vi "Read Output.vi"(0 "VISA resource name":refnum<visa-resource-name>, 7 "Reading Source (T:Voltage)":bool=TRUE, 11 "error in (no error)":errorcluster) -> (4 "VISA resource name out":refnum<visa-resource-name>, 8 "Display Reading":dbl format="%^.4e", 15 "error out":errorcluster)   [LabVIEW 2020, in "Stanford Research PS300 Series.lvlib"]
doc: "This VI reads and displays the current value that is being outputted by the instrument."
uses:
  Stanford Research PS300 Series.lvlib
panel:
  # "Voltage \nCurrent"
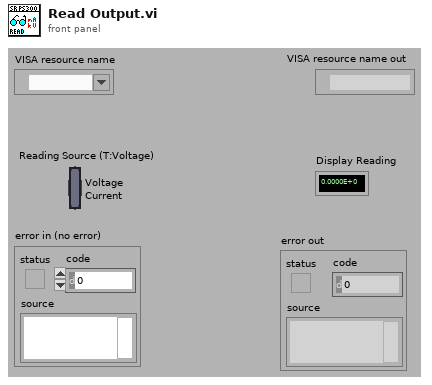
[diagram p1: front panel]
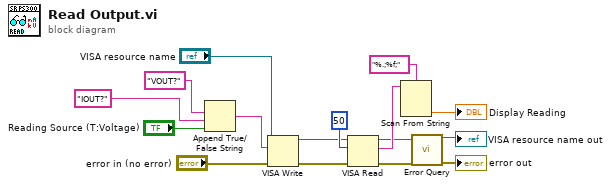
[diagram p0: block diagram]
diagram:
  n1 = Append True/False String(1:"Reading Source (T:Voltage)", 2:"IOUT?" ("false string"), 3:"VOUT?" ("true string")) -> (0:w10:string)  [unwired: 1 in]
  n2 = VISA Write(VISA resource name="VISA resource name", write buffer=w10, error in (no error)="error in (no error)") -> (VISA resource name out=w8:refnum<visa-resource-name>, error out=w7:errorcluster)  [unwired: 1 out]
  n3 = VISA Read(VISA resource name=w8, byte count=u32 50 ("byte count (0)"), error in (no error)=w7) -> (VISA resource name out=w4:refnum<visa-resource-name>, read buffer=w16:string, error out=w3:errorcluster)  [unwired: 1 out]
  n4 = Scan From String(format string="%.;%f;", input string=w16) -> (output 1=→"Display Reading":dbl)  [unwired: 3 in, 3 out]
  n5 = call "Error Query.vi"("VISA resource name"=w4, "error in (no error)"=w3) -> ("VISA resource name out"=→"VISA resource name out":refnum<visa-resource-name>, "error out"=→"error out":errorcluster)  [unwired: 10 in, 2 out]
